vi "VectorToPoint.vi"(1 "Vector":cluster{"x":dbl, "y":dbl, "angle":dbl}) -> (0 "Point":cluster{"x":dbl, "y":dbl})   [LabVIEW 2015, in "Navigation2017.lvlib" / "Util - Navigation2017.lvlib"]
doc: "Converts a vector cluster with an angle to a bare point."
uses:
  Util - Navigation2017.lvlib
panel:
  # "Converts a vector cluster with an angle to a bare point."
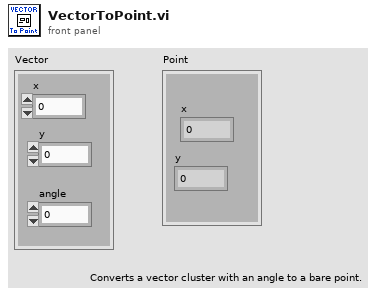
[diagram p1: front panel]
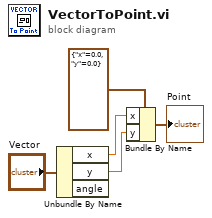
[diagram p0: block diagram]
diagram:
  n1 = Unbundle By Name("Vector") -> ("x"=w3:dbl, "y"=w2:dbl)  [unwired: 1 out]
  n2 = Bundle By Name(cluster=cluster{"x":dbl, "y":dbl} {"x"=0.0, "y"=0.0}, "x"=w3, "y"=w2) -> (→"Point":cluster{"x":dbl, "y":dbl})
